vi "Main v2.vi"() -> ()   [LabVIEW 2012]
uses:
  <vilib>/Simulation/Scripting/Companion Diagram/SimConfigNode/SimParams.ctl
  <vilib>/Simulation/Scripting/Companion Diagram/SimConfigNode/_simSolvers.ctl
  <vilib>/Simulation/Implementation/Shared/SIMSCR Execution Mode.ctl
  <vilib>/Platform/TimedLoop/XDataNode/timing_clust.ctl
  <vilib>/Platform/TimedLoop/XDataNode/nitl_modes.ctl
  <vilib>/Platform/TimedLoop/XDataNode/wakeup.ctl
  <vilib>/Simulation/Param Hierarchy/Typedefs/SIMPH Param Control Actions.ctl
  <vilib>/Simulation/Implementation/Shared/NILVSim_ParamChanged.vi
  <vilib>/Simulation/Implementation/Shared/NILVSim_FinishedLate.vi
  <vilib>/Simulation/Utility/Implementation/SIM Halt.vi
  <vilib>/Simulation/Implementation/Shared/NILVSim_Manager.vi
  <vilib>/Simulation/Implementation/Shared/NILVSim_FinalizeModel.vi
  <vilib>/Simulation/Implementation/Shared/SIM Unbundle Sim Info.vi
  <vilib>/Utility/error.llb/Clear Errors.vi
  <vilib>/Simulation/Implementation/Shared/NILVSim_GetModelError.vi
  <vilib>/Simulation/Implementation/Shared/SIM Bundle Sim Info.vi
  <vilib>/Simulation/Implementation/Shared/SIMSH Read Queue.vi
  <vilib>/Simulation/Implementation/Shared/NILVSim_Initialize.vi
  Unibot/Unibot - State Machine Controller v2.vi
  FPGA IO SubVIs/FPGA RoboteQ Driver.vi
  <vilib>/Simulation/Utility/Implementation/NILVSim Get Time and IsAcceptedStep.vi
  <vilib>/Simulation/Scripting/Companion Diagram/SimConfigNode/SimDog.xnode
  <vilib>/Platform/TimedLoop/XDataNode/XDataNode.xnode
  <vilib>/Simulation/Implementation/XNodeFramework/SimXNode/SimX.xnode
  <vilib>/Platform/TimedLoop/XDataNode/XDNodeRunTimeDep.lvlib
  <vilib>/Simulation/Implementation/Shared/NI_SIM_Implementation.lvlib
panel:
  in  "Tab Control":enum32{"IMU", "Control", "Status", "Errors"}(tab)
  in  "IMU VISA":refnum<visa-resource-name>="ASRL1::INSTR"
  in  "PID gains":T1={"proportional gain (Kc)"=30.0, "integral time (Ti, min)"=0.0, "derivative time (Td, min)"=0.0} {"derivative time (Td, min)" format="%.3f"; "integral time (Ti, min)" format="%.3f"; "proportional gain (Kc)" format="%.3f"}
  in  "Setpoint":dbl(knob) scale=-1.0..1.0
  out "States":dbl[](array[numeric])
  in  "Parameters":T2={"Limit"=10.0, "Control Dead Band"=10.0, "Error Dead Band"=0.0}
  out "Read Loop Count":i32
  out "Received array Size":i32
  out "Processing Loop Count":i32
  out "Command to Serial":string
  out "timed out?":bool
  out "Serial Settings:Number of Bytes at Serial Port":u32
  out "Byte Count":u32
  out "IMU Rean Error":errorcluster
  in  "Error In":errorcluster
  out "RoboteQ Error":errorcluster
  out "Error Out":errorcluster
  in  "stop?":bool
  out "Roll":dbl(knob) scale=-20.0..20.0
  out "Status":string="Kill"
  in  "Kill":bool
  in  "Enable":bool
  out "Top Motor Effort":dbl(knob) scale=-1000.0..1000.0
  out "Bottom Motor Effort":dbl(knob) scale=-1000.0..1000.0
  in  "Mode":T3(ring)
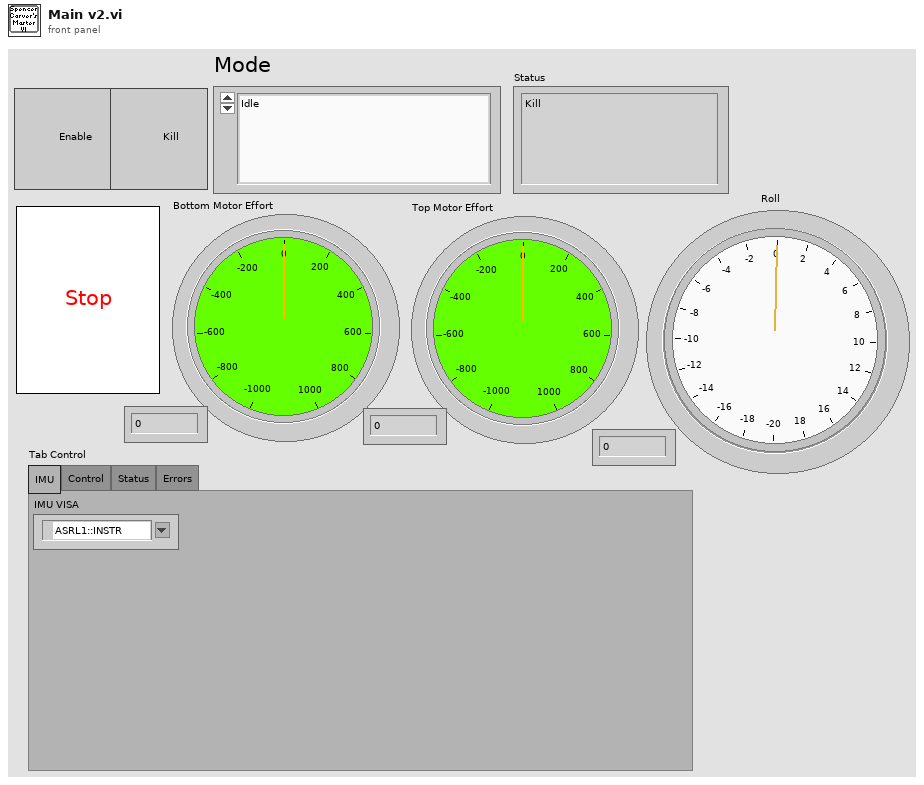
[diagram p1: front panel]
types:
  T1 = cluster{"proportional gain (Kc)":dbl, "integral time (Ti, min)":dbl, "derivative time (Td, min)":dbl}
  T2 = cluster{"Limit":dbl, "Control Dead Band":dbl, "Error Dead Band":dbl}
  T3 = enum16{"Idle", "Linear Balance", "Proportional Balance", "PID Balance", "Emergency"}
  T4 = typedef "901x DMA FPGA Reference.ctl" = refnum<k20>
  T5 = typedef "SIMSCR Execution Mode.ctl" = enum16{"Simulate to Completion", "Single Time-Step Simulation (Fixed Step Only)"}
  T6 = typedef "XDNodeRunTimeDep.lvlib/timing_clust.ctl" = cluster{"Expected End [f-1]":u64, "Actual End [f-1]":u64, "Finished Late? [f-1]":bool, "Expected End [i-1]":u64, "Actual End [i-1]":u64, "Finished Late? [i-1]":bool, "Expected Start [i]":u64, "Actual Start [i]":u64, "Expected Start [f]":u64, "Actual Start [f]":u64, "Source Name":string, "Structure Name":string, "Period":i64, "Deadline":i64, "Offset":i64, "Start":i64, "Priority":i32, "Timeout":i32, "Mode":T7, "Wakeup Reason":T8, "Error":errorcluster, "Source Type":string, "Secondary Source Type":string, "Global End Time":u64, "Global Start Time":u64, "Frame Duration":u64, "Iteration Duration":u64, "Assigned CPU":i32, "I/O Scan Engine Mode":u32}
  T7 = typedef "XDNodeRunTimeDep.lvlib/nitl_modes.ctl" = enum32{"No Change", "Process missed periods, maintain original phase", "Discard missed periods, maintain original phase", "Process missed periods, ignore original phase", "Discard missed periods, ignore original phase"}
  T8 = typedef "XDNodeRunTimeDep.lvlib/wakeup.ctl" = enum32{"Normal", "Aborted", "Asynchronous wakeup", "Timing source error", "Timed loop error", "Timeout"}
  T9 = typedef "SIMPH Param Control Actions.ctl" = enum16{"get params", "set params"}
  T10 = typedef "SimParams.ctl" = cluster{"Initial Time (s)":dbl, "Final Time (s)":dbl, "Step Size (s)":dbl, "ODE Solver":T11, "Minimum Step Size (s)":dbl, "Maximum Step Size (s)":dbl, "Relative Tolerance":dbl, "Absolute Tolerance":dbl, "Software Timing":bool, "Initial Step Size (s)":dbl, "Automatic Fixed Step Size?":bool, "Automatic Discrete Step Size?":bool, "Discrete Step Size (s)":dbl, "Calculate using Time Step":bool, "Solver Wired?":bool, "Prev.Frm.Expected End":u64, "Prev.Frm.Actual End":u64, "Prev.Frm.Finished Late?":bool, "Prev.Iter.Expected End":u64, "Prev.Iter.Actual End":u64, "Prev.Iter.Finished Late?":bool, "Expected Iteration Start":u64, "Actual Iteration Start":u64, "Expected Frame Start":u64, "Actual Frame Start":u64, "Source Name":string, "Name":string, "Period":i64, "Deadline":i64, "Offset":i64, "Start":i64, "Priority":i32, "Timeout":i32, "Processor":i32, "Mode":enum32{"No Change", "Process missed periods, maintain original phase", "Discard missed periods, maintain original phase", "Process missed periods, ignore original phase", "Discard missed periods, ignore original phase"}, "Wakeup reason":enum32{"Normal", "Aborted", "Asynchronous wakeup", "Timing source error", "Timed loop error", "Timeout"}, "Error":errorcluster, "Source Type":string, "Secondary Source Type":string, "Global End Time":u64, "Global Start Time":u64, "Full Solver Reset":bool, "Execution Mode":T5, "Nan/Inf Check":bool, "Custom Solver Library":string, "Solver Is Variable":bool, "custom solver name":string, "Signal Collection Decimation":u32}
  T11 = typedef "_simSolvers.ctl" = enum16{"Runge-Kutta 1 (Euler)", "Runge-Kutta 2", "Runge-Kutta 3", "Runge-Kutta 4", "Runge-Kutta 23 (variable)", "Runge-Kutta 45 (variable)", "BDF (variable)", "Adams-Moulton (variable)", "Rosenbrock (variable)", "Discrete States Only", "SDIRK 4 (variable)", "Radau 5 (variable)", "Radau 9 (variable)", "Radau 13 (variable)", "Radau [Variable Order] (variable)", "Gear's Method (variable)", "Linearizer", "State Query", "Trim Eval", "Custom Solver"}
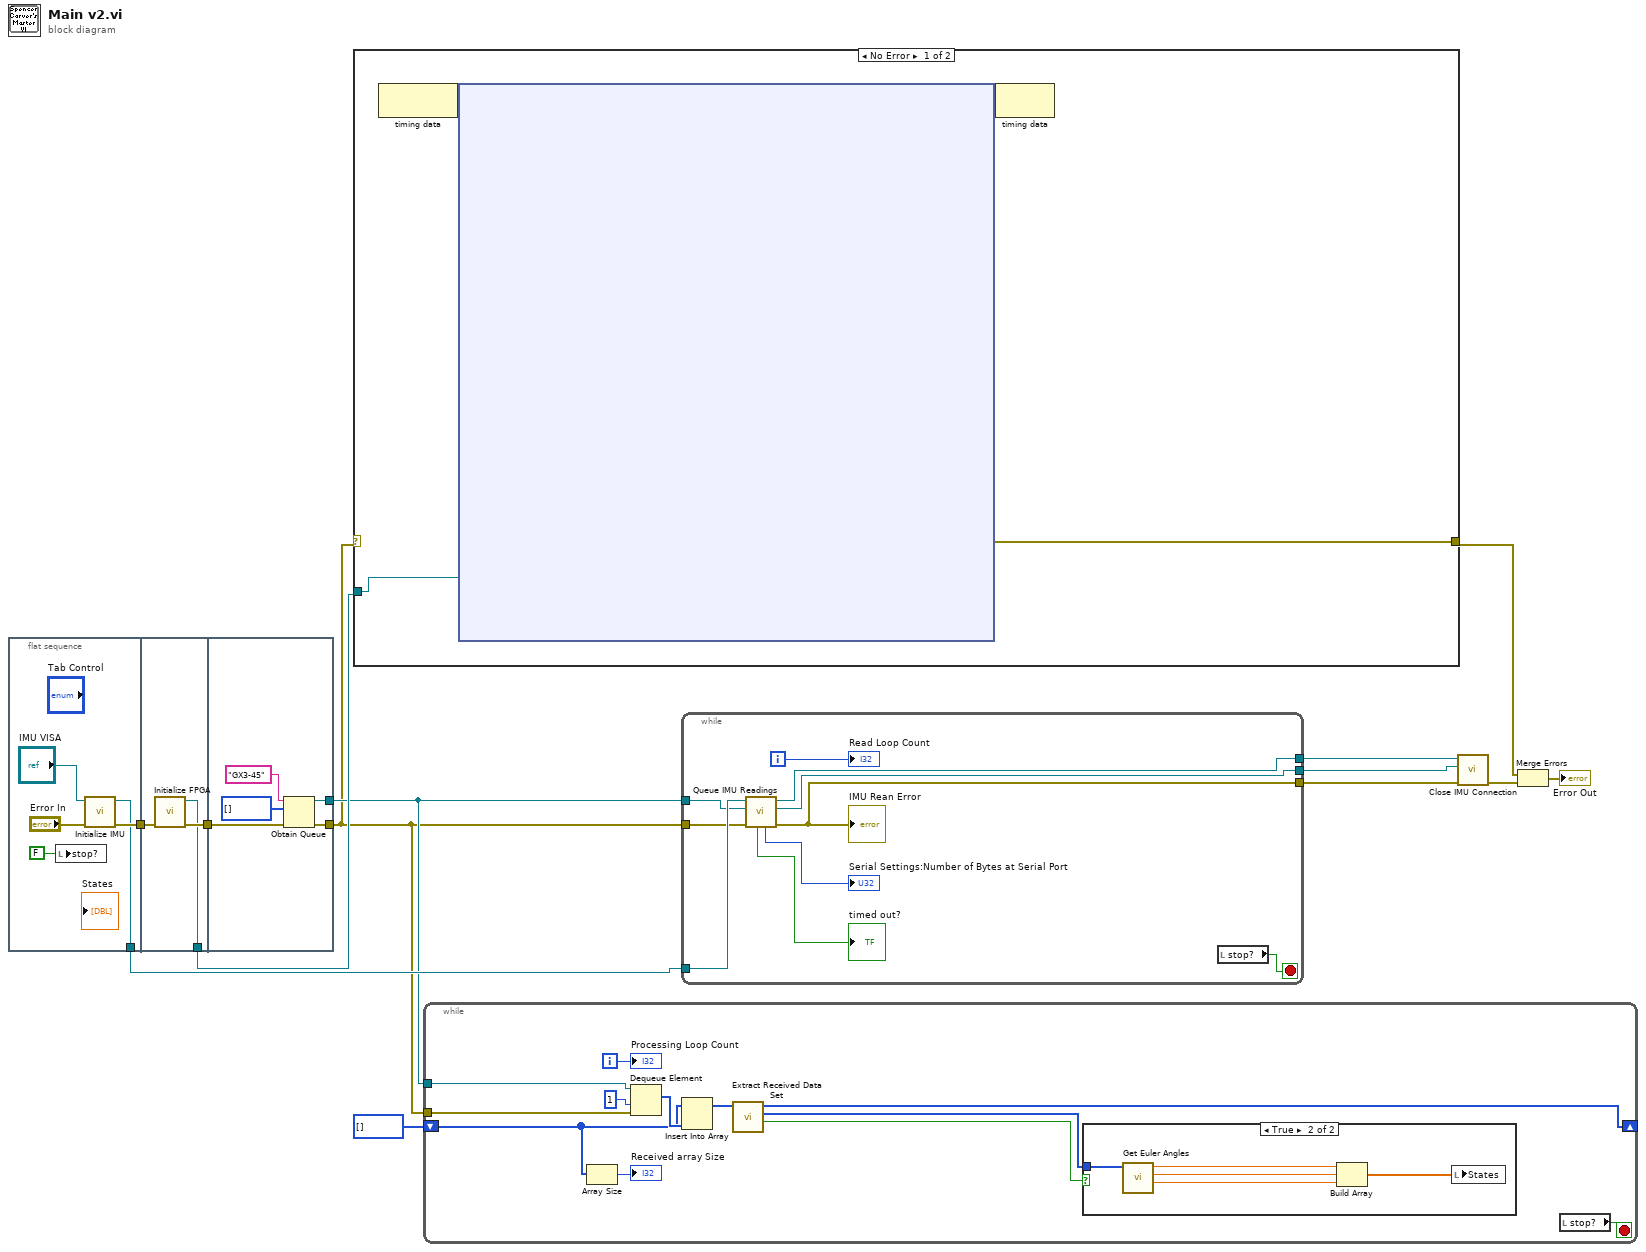
[diagram p0: block diagram]
diagram:
  n1 = flat-sequence {
    tunnel: [w16] -> w6
    tunnel: [w15] -> w3
    tunnel: w6 -> [w21]
    tunnel: [w20] -> w5
    tunnel: [w19] -> w4
    tunnel: w5 -> [w24]
    tunnel: [w23] -> w2
    tunnel: [w22] -> w1
    frame #0 {
      n2 = local write "stop?"(FALSE ("stop?")) -> ()
      n3 = call "Initialize IMU.vi"("error in (no error)"="Error In", "IMU VISA"="IMU VISA") -> ("error out"=w16:errorcluster, "VISA resource name out"=w15:refnum<visa-resource-name>)  [unwired: 8 in]
    }
    frame #1 {
      n4 = call "Initialize FPGA.vi"("error in"=w21) -> ("error out"=w20:errorcluster, "FPGA Out"=w19:T4)  [unwired: 9 in]
    }
    frame #2 {
      n5 = Obtain Queue(name (unnamed)="GX3-45", element data type=u8[] [] ("unsigned byte array"), error in (no error)=w24) -> (queue out=w23:refnum<queue>, error out=w22:errorcluster)  [unwired: 2 in, 1 out]
    }
  }
  n6 = case shown="No Error" w1 {
    selector: w1 -> [_ w348]
    tunnel: [w27 w348] -> w9
    tunnel: w4 -> [w28 _]
    frame No Error {
      n7 = node-c288() -> (w30:variant)  [unwired: 1 out]
      n8 = node-c254 ("Simulation Loop 3")(w30, w28) -> (w29:variant, w27:errorcluster)
      n9 = node-c288(w29) -> ()  [unwired: 1 out]
    }
    frame Error {
    }
  }
  n10 = while {
    shift-right: [w352] -> _
    shift-left: u8[] [] ("element") -> [w356]
    tunnel: w2 -> [w351]
    tunnel: w1 -> [w350]
    i -> [w359]
    stop <- w349 stop-if-true
    n11 = Array Size(array=w356) -> (size(s)=→"Received array Size":i32)
    n12 = Dequeue Element(queue=w351, timeout in ms (-1)=1, error in (no error)=w350) -> (element=w360:u8[])  [unwired: 3 out]
    n13 = Insert Into Array(array=w356, new element=w360) -> (w358:u8[])  [unwired: 1 in]
    n14 = call "Extract Received Data Set.vi"("Received Array In"=w358) -> ("New Data Set Received"=w354:bool, "Extracted Data Set"=w353:u8[], "Received Array Out"=w352:u8[])  [unwired: 7 in, 1 out]
    n15 = case shown="True" w354 {
      tunnel: w353 -> [_ w365]
      frame False {
      }
      frame True {
        n16 = call "Get Euler Angles.vi"("Received Array"=w365) -> ("Yaw (deg)"=w363:dbl, "Pitch (deg)"=w362:dbl, "Roll (deg)"=w364:dbl)  [unwired: 7 in]
        n17 = Build Array(w364, w362, w363) -> (w361:dbl[])
        n18 = local write "States"(w361) -> ()
      }
    }
    n19 = local read "stop?"() -> (w349:bool)
    "Processing Loop Count" <- w359
  }
  n20 = while {
    tunnel: [w374] -> w10
    tunnel: [w373] -> w11
    tunnel: [w372] -> w7
    tunnel: w3 -> [w369]
    tunnel: w2 -> [w368]
    tunnel: w1 -> [w367]
    i -> [w375]
    stop <- w366 stop-if-true
    n21 = call "Queue IMU Readings.vi"("error in (no error)"=w367, "queue"=w368, "reference"=w369) -> ("error out"=w373:errorcluster, "queue out"=w372:refnum<queue>, "VISA resource name out"=w374:refnum<visa-resource-name>, "Serial Settings:Number of Bytes at Serial Port"=→"Serial Settings:Number of Bytes at Serial Port":u32, "timed out?"=→"timed out?":bool)  [unwired: 4 in]
    "IMU Rean Error" <- w373
    n22 = local read "stop?"() -> (w366:bool)
    "Read Loop Count" <- w375
  }
  n23 = call "Close IMU Connection.vi"("Error In"=w11, "queue"=w7, "VISA resource name"=w10) -> ("error out"=w13:errorcluster)  [unwired: 8 in]
  n24 = Merge Errors(w9, w13) -> (→"Error Out":errorcluster)
